vi "test-quintic-spline-00.vi"() -> (3 "Test Passed":bool)   [LabVIEW 2019]
uses:
  <vilib>/Rock Robotics/WPI/ThirdParty/JAS_Junk/TrajLib/POSEwCURVATURE.ctl
  <vilib>/Rock Robotics/WPI/ThirdParty/JAS_Junk/TrajLib/POSE2D.ctl
  <vilib>/Rock Robotics/WPI/ThirdParty/JAS_Junk/TrajLib/TRANSLATION2D.ctl
  <vilib>/Rock Robotics/WPI/ThirdParty/JAS_Junk/TrajLib/ROTATION2D.ctl
  <vilib>/Rock Robotics/WPI/ThirdParty/JAS_Junk/TrajLib/Rotation_CreateAngle.vi
  <vilib>/Rock Robotics/WPI/ThirdParty/JAS_Junk/TrajLib/Translation_Create.vi
  <vilib>/Rock Robotics/WPI/ThirdParty/JAS_Junk/TrajLib/Util_CalcDist.vi
  <vilib>/Rock Robotics/WPI/ThirdParty/JAS_Junk/TrajLib/Trajectory_Library.lvlib
panel:
  out "XY Graph":cluster{dbl[], dbl[]}(graph)
  out "Numb\nWaypoints":i32
  out "All Interior \nwayPoints\nFound (True)":bool
  out "end rot = 0":dbl
  out "end y = 0":dbl
  out "end x = 0":dbl
  out "start rot = 0":dbl
  out "start y = 0":dbl
  out "start x = 0":dbl
  out "max dtheta < 0.0872":dbl
  out "max dy < 0.00127":dbl
  out "max dx  < 0.127":dbl
  out "Overall Error":errorcluster
  out "Elements":i32
  out "Create Spline Error":errorcluster
  out "SplinePoses\nWCurve":T1[](array[typedef]) {"POSE"."ROTATION"."SIN" format="%13.4f"; "POSE"."ROTATION"."COS" format="%13.4f"; "POSE"."ROTATION"."VALUE" format="%13.4f"; "POSE"."TRANSLATION"."Y" format="%14.3f"; "POSE"."TRANSLATION"."X" format="%14.3f"}
  out "Elapsed Time":dbl
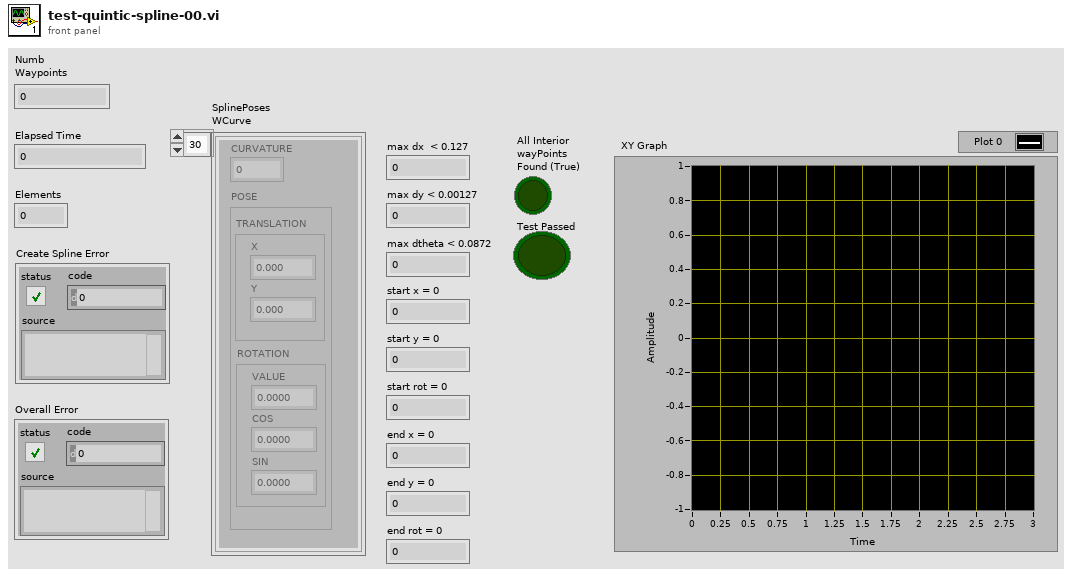
[diagram p1: front panel]
types:
  T1 = typedef "Trajectory_Library.lvlib/POSEwCURVATURE.ctl" = cluster{"CURVATURE":dbl, "POSE":T2}
  T2 = typedef "Trajectory_Library.lvlib/POSE2D.ctl" = cluster{"TRANSLATION":T3, "ROTATION":T4}
  T3 = typedef "Trajectory_Library.lvlib/TRANSLATION2D.ctl" = cluster{"X":dbl, "Y":dbl}
  T4 = typedef "Trajectory_Library.lvlib/ROTATION2D.ctl" = cluster{"VALUE":dbl, "COS":dbl, "SIN":dbl}
  T5 = typedef "Trajectory_Library.lvlib/SPLINE_CTRL_VECTOR.ctl" = cluster{"Xs":dbl[], "Ys":dbl[]}
  T6 = typedef "Trajectory_Library.lvlib/SPLINE.ctl" = cluster{"Degree":i32, "Coefficients":T7}
  T7 = typedef "NI_Matrix.lvlib/RealMatrix.ctl" = dbl[][]
  T8 = typedef "Trajectory_Library.lvlib/TWIST2D.ctl" = cluster{"dX":dbl, "dY":dbl, "dTHETA":dbl}
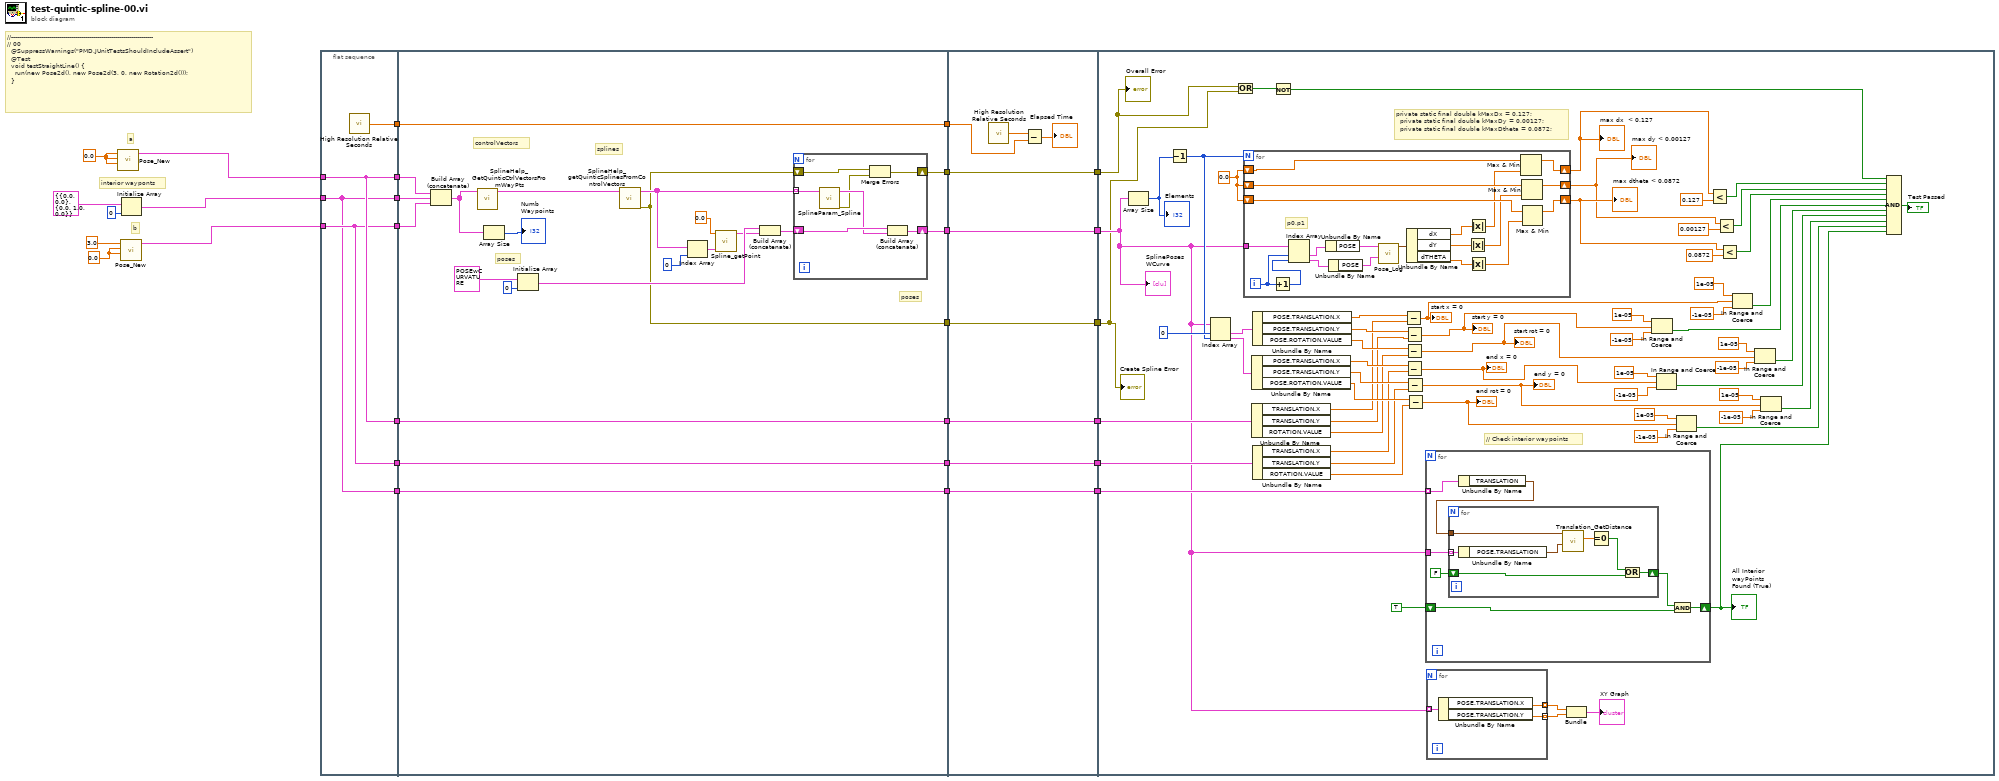
[diagram p0: block diagram]
diagram:
  w26 = 0.0 ("Y")
  w28 = 0.0 ("X")
  # "interior wayponts"
  # "b"
  # "a"
  # "//-----------------------------------------------------------------------\n// 00\n  @SuppressWarnings(\"PMD.JUnitTestsShouldIncludeAssert\")\n  @Test\n  void testStraightLine() {\n    run(new Pose2d(), new Pose2d(3, 0, new Rotation2d()));\n  }"
  n1 = call <vilib>:"Pose_New.vi"("Heading"=w28, "Y"=w28, "X"=w28) -> ("out POSe"=w25:T2)  [unwired: 8 in]
  n2 = call <vilib>:"Pose_New.vi"("Heading"=w26, "Y"=w26, "X"=3.0) -> ("out POSe"=w23:T2)  [unwired: 8 in]
  n3 = Initialize Array(T2 {"TRANSLATION"={"X"=0.0, "Y"=0.0}, "ROTATION"={"VALUE"=0.0, "COS"=1.0, "SIN"=0.0}} ("POSE"), 0 ("dimension size")) -> (w2:T2[])
  n4 = flat-sequence {
    tunnel: w25 -> [w31]
    tunnel: [w31] -> w24
    tunnel: w23 -> [w30]
    tunnel: [w30] -> w22
    tunnel: [w32] -> w21
    tunnel: [w31] -> w13
    tunnel: [w30] -> w10
    tunnel: [w29] -> w5
    tunnel: w2 -> [w29]
    tunnel: [w29] -> w1
    tunnel: w24 -> [w38]
    tunnel: w22 -> [w36]
    tunnel: [w54] -> w20
    tunnel: w21 -> [w54]
    tunnel: [w44] -> w19
    tunnel: [w43] -> w17
    tunnel: [w42] -> w15
    tunnel: w13 -> [w41]
    tunnel: [w41] -> w12
    tunnel: w10 -> [w40]
    tunnel: [w40] -> w9
    tunnel: [w39] -> w6
    tunnel: w5 -> [w39]
    tunnel: w1 -> [w35]
    tunnel: w20 -> [w70]
    tunnel: w19 -> [w69]
    tunnel: [w69] -> w18
    tunnel: w17 -> [w68]
    tunnel: [w68] -> w16
    tunnel: w15 -> [w67]
    tunnel: [w67] -> w14
    tunnel: w12 -> [w64]
    tunnel: [w64] -> w11
    tunnel: w9 -> [w63]
    tunnel: [w63] -> w8
    tunnel: [w62] -> w7
    tunnel: w6 -> [w62]
    tunnel: w18 -> [w111]
    tunnel: w16 -> [w98]
    tunnel: w14 -> [w97]
    tunnel: w11 -> [w133]
    tunnel: w8 -> [w132]
    tunnel: w7 -> [w115]
    frame #0 {
      n5 = call <vilib>:"High Resolution Relative Seconds.vi"() -> ("relative seconds"=w32:dbl)
    }
    frame #1 {
      # "poses"
      # "poses"
      # "splines"
      # "controlVectors"
      n6 = Build Array (concatenate)(w38, w35, w36) -> (w34:T2[])
      n7 = call <vilib>:"SplineHelp_GetQuinticCtrlVectorsFromWayPts.vi"("WayPoints"=w34) -> ("SplineControlVectors"=w37:T5[])  [unwired: 10 in]
      n8 = Array Size(array=w34) -> (size(s)=→"Numb\nWaypoints":i32)
      n9 = Initialize Array(T1 {"CURVATURE"=0.0, "POSE"={"TRANSLATION"={"X"=0.0, "Y"=0.0}, "ROTATION"={"VALUE"=0.0, "COS"=1.0, "SIN"=0.0}}} ("POSEwCURVATURE"), 0 ("dimension size")) -> (w48:T1[])
      n10 = call <vilib>:"SplineHelp_getQuinticSplinesFromControlVectors.vi"("ControlVectors"=w37) -> ("error out"=w43:errorcluster, "splines"=w45:T6[])  [unwired: 9 in]
      n11 = Index Array(array=w45, index=0) -> (element=w50:T6)
      n12 = call <vilib>:"Spline_getPoint.vi"("inputSPLINE"=w50, "Time"=0.0) -> ("POSEwCURVATURE"=w47:T1)  [unwired: 9 in]
      n13 = Build Array (concatenate)(w48, w47) -> (w46:T1[])
      n14 = for {
        shift-right: [w58] -> w44
        shift-left: w46 -> [w60]
        tunnel: w45 -> [w61] mode=indexing
        shift-right: [w56] -> w42
        shift-left: w43 -> [w57]
        n15 = call <vilib>:"SplineParam_Spline.vi"("inputSPLINE"=w61) -> ("error out"=w55:errorcluster, "outputPOSEwCURVATURE"=w59:T1[])  [unwired: 9 in]
        n16 = Merge Errors(w57, w55) -> (w56:errorcluster)
        n17 = Build Array (concatenate)(w60, w59) -> (w58:T1[])
      }
    }
    frame #2 {
      n18 = call <vilib>:"High Resolution Relative Seconds.vi"() -> ("relative seconds"=w65:dbl)
      n19 = Subtract(x=w65, y=w70) -> (x-y=→"Elapsed Time":dbl)
    }
    frame #3 {
      w134 = 0.0
      # "// Check interior waypoints"
      # "private static final double kMaxDx = 0.127;\n  private static final double kMaxDy = 0.00127;\n  private static final double kMaxDtheta = 0.0872;"
      n20 = Array Size(array=w111) -> (size(s)=w135:i32)
      "Elements" <- w135
      n21 = Decrement(x=w135) -> (x-1=w130:i32)
      n22 = Index Array(array=w111, index #1=0 ("index"), index #2=w130) -> (element #1=w129:T1, element #2=w128:T1)
      n23 = Or(x=w97, y=w98) -> (x .or. y?=w99:bool)
      n24 = for {
        N: w130 -> [_]
        tunnel: w111 -> [w170]
        shift-right: [w161] -> w103
        shift-left: w134 -> [w158]
        shift-right: [w159] -> w105
        shift-left: w134 -> [w156]
        shift-right: [w160] -> w104
        shift-left: w134 -> [w157]
        i -> [w172]
        # "p0,p1"
        n25 = Increment(x=w172) -> (x+1=w171:i32)
        n26 = Index Array(array=w170, index #1=w172, index #2=w171) -> (element #1=w169:T1, element #2=w168:T1)
        n27 = Unbundle By Name(w169) -> ("POSE"=w167:T2)
        n28 = Unbundle By Name(w168) -> ("POSE"=w166:T2)
        n29 = call <vilib>:"Pose_Log.vi"("end POSE"=w166, "in POSE"=w167) -> ("out TWIST"=w165:T8)  [unwired: 9 in]
        n30 = Unbundle By Name(w165) -> ("dX"=w162:dbl, "dY"=w163:dbl, "dTHETA"=w164:dbl)
        n31 = Absolute Value(x=w163) -> (abs(x)=w154:dbl)
        n32 = Absolute Value(x=w162) -> (abs(x)=w155:dbl)
        n33 = Absolute Value(x=w164) -> (abs(x)=w153:dbl)
        n34 = Max & Min(x=w158, y=w155) -> (max(x,y)=w161:dbl)  [unwired: 1 out]
        n35 = Max & Min(x=w157, y=w154) -> (max(x,y)=w160:dbl)  [unwired: 1 out]
        n36 = Max & Min(x=w156, y=w153) -> (max(x,y)=w159:dbl)  [unwired: 1 out]
      }
      "max dx  < 0.127" <- w103
      "max dy < 0.00127" <- w104
      "max dtheta < 0.0872" <- w105
      n37 = Unbundle By Name(w128) -> ("POSE.TRANSLATION.X"=w124:dbl, "POSE.TRANSLATION.Y"=w123:dbl, "POSE.ROTATION.VALUE"=w122:dbl)
      n38 = Unbundle By Name(w133) -> ("TRANSLATION.X"=w121:dbl, "TRANSLATION.Y"=w120:dbl, "ROTATION.VALUE"=w119:dbl)
      n39 = Unbundle By Name(w129) -> ("POSE.TRANSLATION.X"=w127:dbl, "POSE.TRANSLATION.Y"=w126:dbl, "POSE.ROTATION.VALUE"=w125:dbl)
      n40 = Unbundle By Name(w132) -> ("TRANSLATION.X"=w118:dbl, "TRANSLATION.Y"=w117:dbl, "ROTATION.VALUE"=w116:dbl)
      n41 = Not(x=w99) -> (.not. x?=w96:bool)
      n42 = Subtract(x=w127, y=w121) -> (x-y=w92:dbl)
      "start x = 0" <- w92
      n43 = Subtract(x=w126, y=w120) -> (x-y=w71:dbl)
      "start y = 0" <- w71
      n44 = Subtract(x=w125, y=w119) -> (x-y=w75:dbl)
      "start rot = 0" <- w75
      n45 = Subtract(x=w124, y=w118) -> (x-y=w76:dbl)
      "end x = 0" <- w76
      n46 = Subtract(x=w123, y=w117) -> (x-y=w83:dbl)
      "end y = 0" <- w83
      n47 = Subtract(x=w122, y=w116) -> (x-y=w87:dbl)
      "end rot = 0" <- w87
      n48 = for {
        tunnel: w115 -> [w140] mode=indexing
        tunnel: w111 -> [w145]
        shift-right: [w144] -> w95
        shift-left: TRUE -> [w143]
        n49 = Unbundle By Name(w140) -> ("TRANSLATION"=w139:T3)
        n50 = for {
          tunnel: w145 -> [w149] mode=indexing
          shift-right: [w152] -> w141
          shift-left: FALSE -> [w151]
          tunnel: w139 -> [w150]
          n51 = Unbundle By Name(w149) -> ("POSE.TRANSLATION"=w148:T3)
          n52 = call <vilib>:"Translation_GetDistance.vi"("other Translation"=w148, "In Translation"=w150) -> ("Distance"=w147:dbl)  [unwired: 9 in]
          n53 = Equal To 0?(x=w147) -> (x = 0?=w146:bool)
          n54 = Or(x=w146, y=w151) -> (x .or. y?=w152:bool)
        }
        n55 = And(x=w141, y=w143) -> (x .and. y?=w144:bool)
      }
      "All Interior \nwayPoints\nFound (True)" <- w95
      n56 = for {
        tunnel: [w138] -> w113 mode=indexing
        tunnel: [w137] -> w112 mode=indexing
        tunnel: w111 -> [w136] mode=indexing
        n57 = Unbundle By Name(w136) -> ("POSE.TRANSLATION.X"=w138:dbl, "POSE.TRANSLATION.Y"=w137:dbl)
      }
      n58 = Bundle(w113, w112) -> (→"XY Graph":cluster{dbl[], dbl[]})  [unwired: 1 in]
      n59 = In Range and Coerce(upper limit=1e-05, x=w71, lower limit=-1e-05) -> (In Range?=w72:bool)  [unwired: 1 out]
      n60 = In Range and Coerce(upper limit=1e-05, x=w76, lower limit=-1e-05) -> (In Range?=w78:bool)  [unwired: 1 out]
      n61 = In Range and Coerce(upper limit=1e-05, x=w87, lower limit=-1e-05) -> (In Range?=w88:bool)  [unwired: 1 out]
      n62 = Less?(x=w103, y=0.127) -> (x < y?=w102:bool)
      n63 = Less?(x=w104, y=0.00127) -> (x < y?=w101:bool)
      n64 = Less?(x=w105, y=0.0872) -> (x < y?=w100:bool)
      n65 = In Range and Coerce(upper limit=1e-05, x=w92, lower limit=-1e-05) -> (In Range?=w91:bool)  [unwired: 1 out]
      n66 = In Range and Coerce(upper limit=1e-05, x=w75, lower limit=-1e-05) -> (In Range?=w77:bool)  [unwired: 1 out]
      n67 = In Range and Coerce(upper limit=1e-05, x=w83, lower limit=-1e-05) -> (In Range?=w84:bool)  [unwired: 1 out]
      n68 = Compound Arithmetic op=AND(w96, w102, w101, w100, w91, w72, w77, w78, w84, w88, w95) -> (→"Test Passed":bool)
      "SplinePoses\nWCurve" <- w111
      "Create Spline Error" <- w98
      "Overall Error" <- w97
    }
  }
